vi "c_ctre_phoenix6_platform_write_string.vi"(0 "String 2":string, 1 "String 4":string, 2 "Numeric 2":dbl) -> (20 "Numeric":i32, 21 "String":string, 22 "String 3":string)   [LabVIEW 2023]
uses:
  <vilib>/Rock Robotics/WPI/ThirdParty/Phoenix-LabVIEW/Controls/DriverLib.ctl
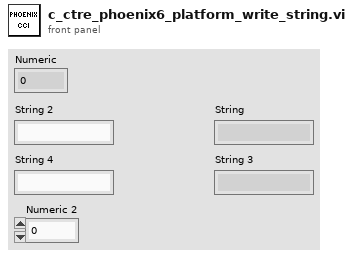
[diagram p1: front panel]
types:
  T1 = typedef "DriverLib.ctl" = path
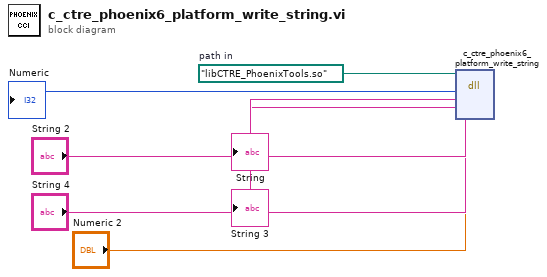
[diagram p0: block diagram]
diagram:
  w7 = T1 path "libCTRE_PhoenixTools.so"  # path in
  n1 = dll-call lib="?" fn="c_ctre_phoenix6_platform_write_string"(path in=w7, "String 2", "String 4", "Numeric 2") -> (→"Numeric":i32, →"String":string, →"String 3":string)  [unwired: 3 in, 2 out]
